vi "Render.vi"(8 "error in (no error)":errorcluster, 11 "XRay Cabinet in":refnum<class "XRay Cabinet.lvclass">) -> (0 "error out":errorcluster, 2 "Scene Object":refnum<vi>, 3 "XRay Cabinet out":refnum<class "XRay Cabinet.lvclass">)   [LabVIEW 2026, in "XRay Cabinet.lvclass"]
uses:
  XRay Cabinet.lvclass
  XRay Cabinet.lvclass/XRay Cabinet.ctl
  <vilib>/picture/3D Picture Control/Object/Add Object (reference).vi
  XRay Scene/XRay Scene.lvclass
  <vilib>/picture/3D Picture Control/NI_3D Picture Control.lvlib
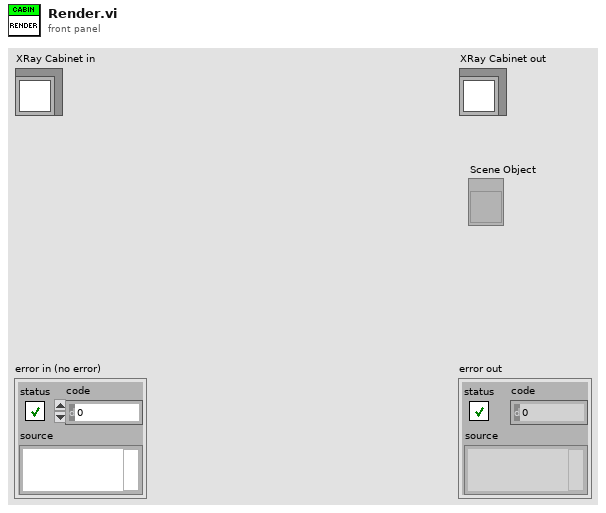
[diagram p1: front panel]
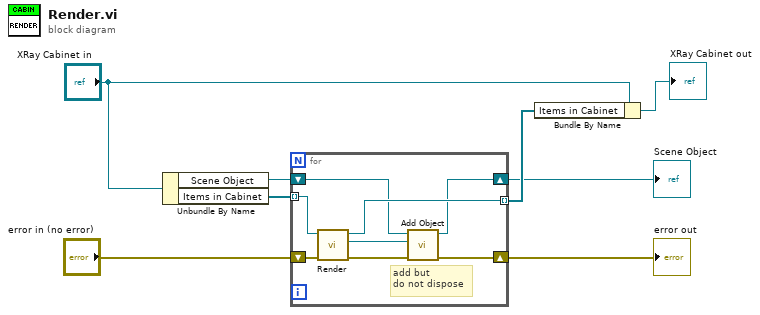
[diagram p0: block diagram]
diagram:
  n1 = Unbundle By Name("XRay Cabinet in") -> ("Scene Object"=w3:refnum<vi>, "Items in Cabinet"=w8:refnum<class "XRay Scene.lvclass">[])
  n2 = for {
    tunnel: w8 -> [w16] mode=indexing
    tunnel: [w15] -> w6 mode=indexing
    shift-right: [w12] -> w4
    shift-left: w3 -> [w13]
    shift-right: [w9] -> w1
    shift-left: "error in (no error)" -> [w14]
    # "add but\ndo not dispose"
    n3 = call-dynamic "Render.vi"("error in (no error)"=w14, "XRay Scene in"=w16) -> ("error out"=w10:errorcluster, "Scene Object"=w11:refnum<vi>, "XRay Scene out"=w15:refnum<class "XRay Scene.lvclass">)  [unwired: 7 in]
    n4 = call-poly <vilib>:"Add Object.vi"("error in (no error)"=w10, "New Object In"=w11, "Scene Object In"=w13) -> ("error out"=w9:errorcluster, "Scene Object Out"=w12:refnum<vi>)  [unwired: 6 in, 1 out]
  }
  "error out" <- w1
  "Scene Object" <- w4
  n5 = Bundle By Name(cluster="XRay Cabinet in", "Items in Cabinet"=w6) -> (→"XRay Cabinet out":refnum<class "XRay Cabinet.lvclass">)
